vi "Read Value.vi"(8 "error in":errorcluster, 11 "Property in":refnum<class "Property.lvclass">) -> (0 "error out":errorcluster, 2 "Value":variant, 3 "Property out":refnum<class "Property.lvclass">)   [LabVIEW 2024, in "Parser.lvlib" / "Property.lvclass"]
uses:
  Property.lvclass
  Property.lvclass/Property.ctl
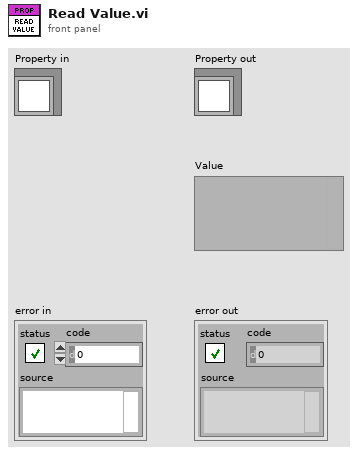
[diagram p1: front panel]
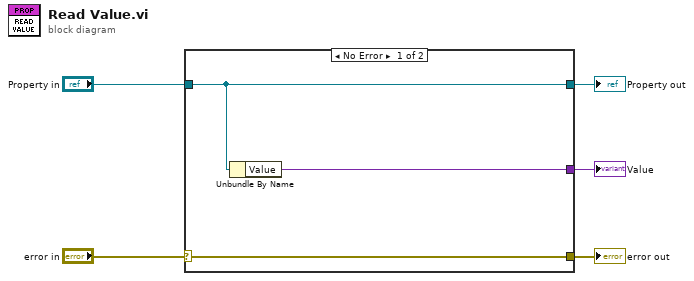
[diagram p0: block diagram]
diagram:
  n1 = case shown="No Error" "error in" {
    selector: "error in" -> [w8 w10]
    tunnel: [w8 w10] -> w4
    tunnel: [w7 w9] -> w2
    tunnel: "Property in" -> [w7 w9]
    tunnel: [w6 _] -> w1
    frame No Error {
      n2 = Unbundle By Name(w7) -> ("Value"=w6:variant)
    }
    frame Error {
    }
  }
  "error out" <- w4
  "Property out" <- w2
  "Value" <- w1
